vi "InstallBookIntoShelf.vi"(1 "FileZipped":string, 3 "Book Name":string) -> (0 "error out":errorcluster)   [LabVIEW 2012]
uses:
  <userlib>/BotSpeak/Devices/EvalRIO/FTPCodes/FTPParameters.ctl
panel:
  in  "Parameters":T1={"Book Folder Name"="", "Full file name"="", "Remote Path"="bookfiles/", "Shelf folder"=path "", "Existing books"=[], "Dialog?"=enum."No Dialog", "New Format?"=FALSE}
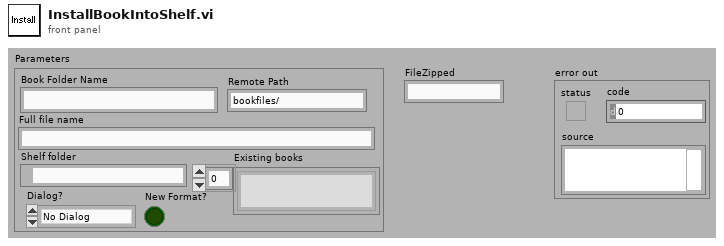
[diagram p1: front panel]
types:
  T1 = typedef "FTPParameters.ctl" = cluster{"Book Folder Name":string, "Full file name":string, "Remote Path":string, "Shelf folder":path, "Existing books":string[], "Dialog?":enum16{"No Dialog", "Dialog", "Overwrite"}, "New Format?":bool}
  T2 = typedef "PathsGlobal.ctl" = cluster{"Root":path, "Shelves":path, "Cmds":path, "Plugins":path}
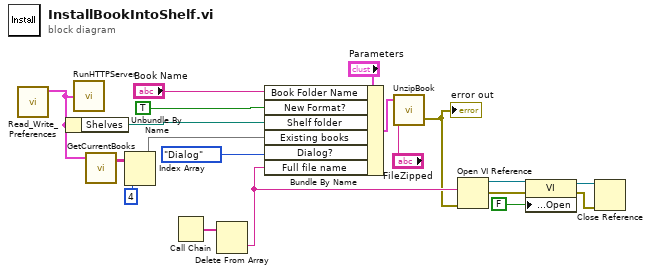
[diagram p0: block diagram]
diagram:
  n1 = call <userlib>:"Read_Write_Preferences.vi"() -> ("Paths"=w11:T2)  [unwired: 1 in, 4 out]
  n2 = Unbundle By Name(w11) -> ("Shelves"=w16:path)
  n3 = call <userlib>:"RunHTTPServer.vi"("Paths"=w11) -> ()
  n4 = call <userlib>:"GetCurrentBooks.vi"("Paths"=w11) -> ("books"=w17:string[][])  [unwired: 2 in, 1 out]
  n5 = Index Array(array=w17, index (col)=4 ("disabled index (col)")) -> (element=w19:string[])  [unwired: 1 in]
  n6 = Call Chain() -> (call chain=w8:string[])
  n7 = Delete From Array(array=w8) -> (deleted portion=w7:string)  [unwired: 2 in, 1 out]
  n8 = Bundle By Name(cluster="Parameters", "Book Folder Name"="Book Name", "New Format?"=TRUE, "Shelf folder"=w16, "Existing books"=w19, "Dialog?"=enum16{"No Dialog", "Dialog", "Overwrite"}."Dialog", "Full file name"=w7) -> (w14:T1)
  n9 = call <userlib>:"UnzipBook.vi"("FileZipped"="FileZipped", "Parameters"=w14) -> ("error out"=w1:errorcluster)  [unwired: 1 in, 1 out]
  "error out" <- w1
  n10 = Open VI Reference(vi path=w7, error in (no error)=w1) -> (vi reference=w6:refnum<vi>, error out=w3:errorcluster)  [unwired: 4 out]
  n11 = property class="VI"(reference=w6, error in=w3, "Front Panel.Open"=FALSE ("Front Panel Window:Open")) -> (reference out=w4:refnum<vi>, error out=w5:errorcluster)
  n12 = Close Reference(reference=w4, error in (no error)=w5) -> ()  [unwired: 1 out]
